vi "Ch1-Ex4.vi"() -> ()   [LabVIEW 2018]
panel:
  out "Array":dbl[](array[numeric])
  out "Waveform Graph":dbl[](graph)
  out "Waveform Chart":dbl(graph)
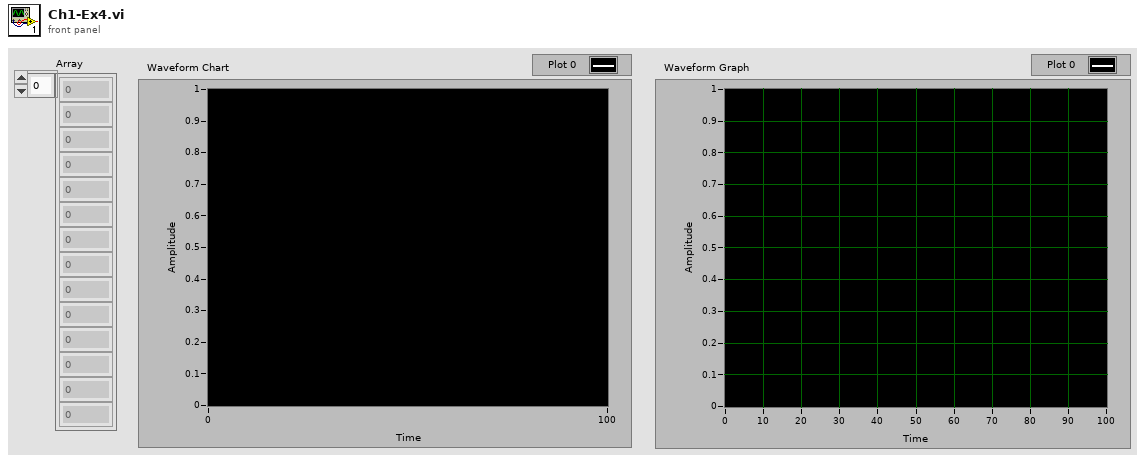
[diagram p1: front panel]
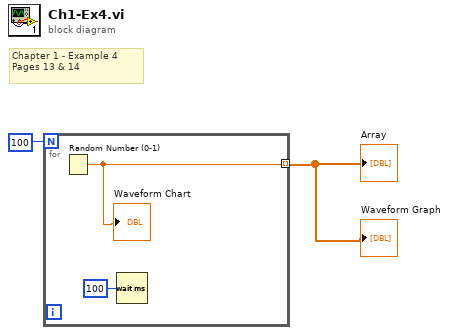
[diagram p0: block diagram]
diagram:
  # "Chapter 1 - Example 4\nPages 13 & 14"
  n1 = for {
    N: 100 -> [_]
    tunnel: [w4] -> w1 mode=indexing
    n2 = Random Number (0-1)() -> (number: 0 to 1=w4:dbl)
    "Waveform Chart" <- w4
    n3 = Wait (ms)(milliseconds to wait=u32 100) -> ()  [unwired: 1 out]
  }
  "Waveform Graph" <- w1
  "Array" <- w1
